vi "Correct_RD_Files.vi"() -> ()   [LabVIEW 2022 SP3]
panel:
  out "error out":errorcluster
  out "Number of strings found":i32
  out "Current File Number":i32
  out "No of Files Changed":i32
  out "Current FIlename":path
  in  "stop":bool
  out "Total Number of Files":i32
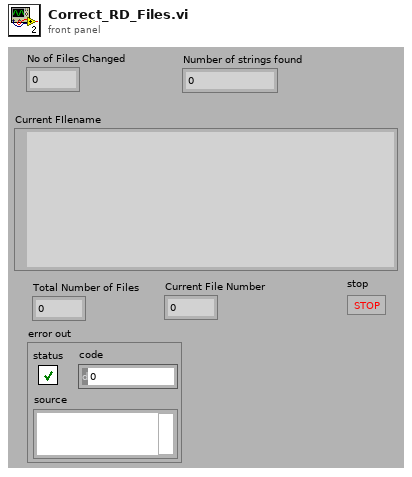
[diagram p1: front panel]
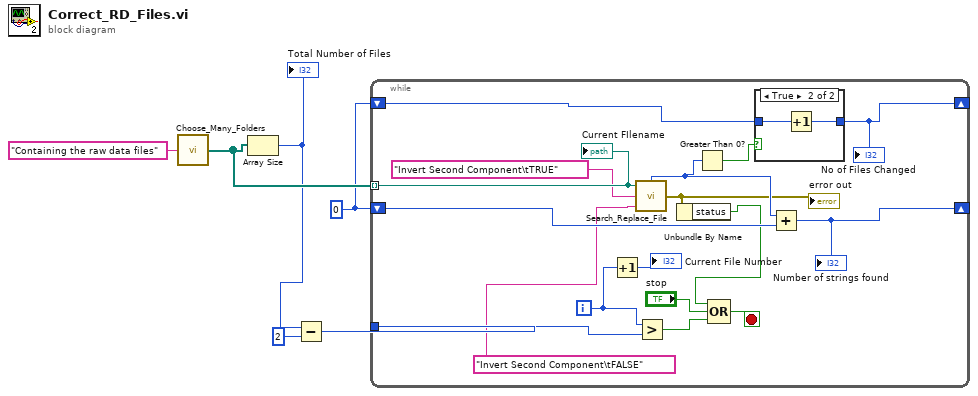
[diagram p0: block diagram]
diagram:
  w2 = 0
  n1 = call "Choose_Many_Folders.vi"("Purpose of choosing folder"="Containing the raw data files") -> ("Files"=w6:path[])
  n2 = Array Size(array=w6) -> (size(s)=w4:i32)
  "Total Number of Files" <- w4
  n3 = Subtract(x=w4, y=2) -> (x-y=w5:i32)
  n4 = while {
    tunnel: w6 -> [w23] mode=indexing
    tunnel: w5 -> [w22]
    shift-right: [w18] -> _
    shift-left: w2 -> [w17]
    shift-right: [w13] -> _
    shift-left: w2 -> [w14]
    i -> [w12]
    stop <- w19 stop-if-true
    n5 = Increment(x=w12) -> (x+1=→"Current File Number":i32)
    n6 = call "Search_Replace_File.vi"("Replace_String"="Invert Second Component\tFALSE", "Search_String"="Invert Second Component\tTRUE", "Path"=w23) -> ("error out"=w10:errorcluster, "Number Found"=w16:i32)
    "error out" <- w10
    n7 = Greater?(x=w12, y=w22) -> (0:w21:bool)
    n8 = Unbundle By Name(w10) -> ("status"=w9:bool)
    n9 = Greater Than 0?(x=w16) -> (x > 0?=w15:bool)
    n10 = Compound Arithmetic op=OR(w9, "stop", w21) -> (w19:bool)
    n11 = case shown="True" w15 {
      tunnel: w14 -> [w24 w26]
      tunnel: [w24 w25] -> w13
      frame False {
      }
      frame True {
        n12 = Increment(x=w26) -> (x+1=w25:i32)
      }
    }
    "No of Files Changed" <- w13
    n13 = Add(x=w16, y=w17) -> (x+y=w18:i32)
    "Number of strings found" <- w18
    "Current FIlename" <- w23
  }
